vi "Move Menu Up.vi"(8 "error in (no error)":errorcluster, 11 "Display State In":T1={"Numeric"=0.0, "Array of Button References"=[], "Space Between Menu Buttons"=0, "Number of Menu Buttons"=0, "Array of Button Names"=[], "Most Recent Vertical Position"=0, "This VI"=refnum, "Current Action"=enum."Not Moving", "Most Recent Distance Traveled"=0, "Method"=enum."Move Up", "Data In"=0} caption="State") -> (0 "error out":errorcluster, 3 "Display State Out":T1={"Numeric"=0.0, "Array of Button References"=[], "Space Between Menu Buttons"=0, "Number of Menu Buttons"=0, "Array of Button Names"=[], "Most Recent Vertical Position"=0, "This VI"=refnum, "Current Action"=enum."Not Moving", "Most Recent Distance Traveled"=0, "Method"=enum."Move Up", "Data In"=0} caption="State")   [LabVIEW 2011, in "Sliding Menu Library.lvlib" / "Sliding Menu XControl.xctl"]
uses:
  Sliding Menu XControl.xctl
  Sliding Menu State.ctl
  Menu Button Library/Menu Button xControl/Menu Button xControl.xctl
  Sliding Menu SubVIs/Sliding Menu Type Definitions/Current User Action.ctl
  Sliding Menu Methods.ctl
  Sliding Menu Data.ctl
  Sliding Menu Library.lvlib
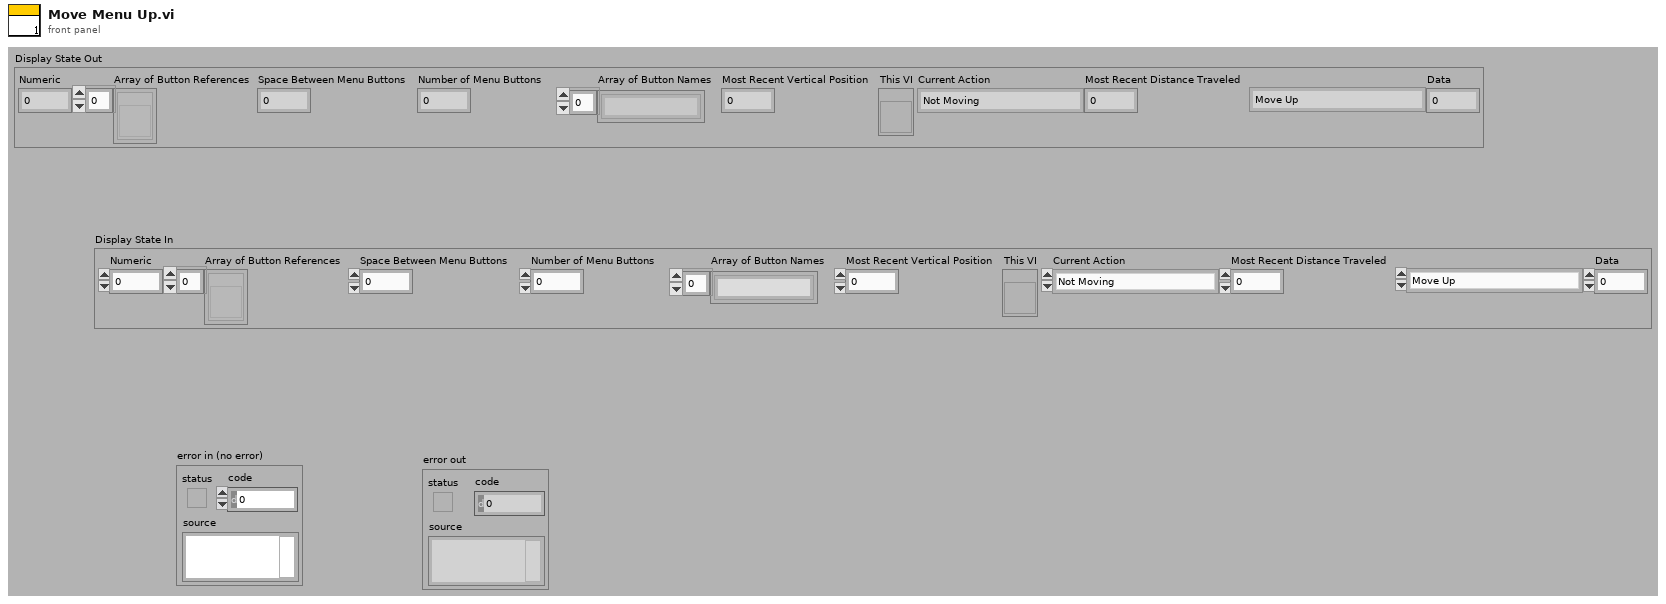
[diagram p1: front panel]
types:
  T1 = typedef "Sliding Menu Library.lvlib/Sliding Menu XControl.xctl/Sliding Menu State.ctl" = cluster{"Numeric":dbl, "Array of Button References":refnum<vi>[], "Space Between Menu Buttons":i32, "Number of Menu Buttons":i32, "Array of Button Names":string[], "Most Recent Vertical Position":i32, "This VI":refnum<vi>, "Current Action":T2, "Most Recent Distance Traveled":i32, "Method":T3, "Data In":T4}
  T2 = typedef "Sliding Menu Library.lvlib/Current User Action.ctl" = enum16{"Not Moving", "Mouse Down", "Mouse Up No Dragging", "Bounce Up Needed", "Bounce Down Needed", "Dragging", "Easing"}
  T3 = typedef "Sliding Menu Methods.ctl" = enum16{"Resize", "Move Up", "Move Down", "Move to 0"}
  T4 = typedef "Sliding Menu Library.lvlib/Sliding Menu XControl.xctl/Sliding Menu Data.ctl" = i32
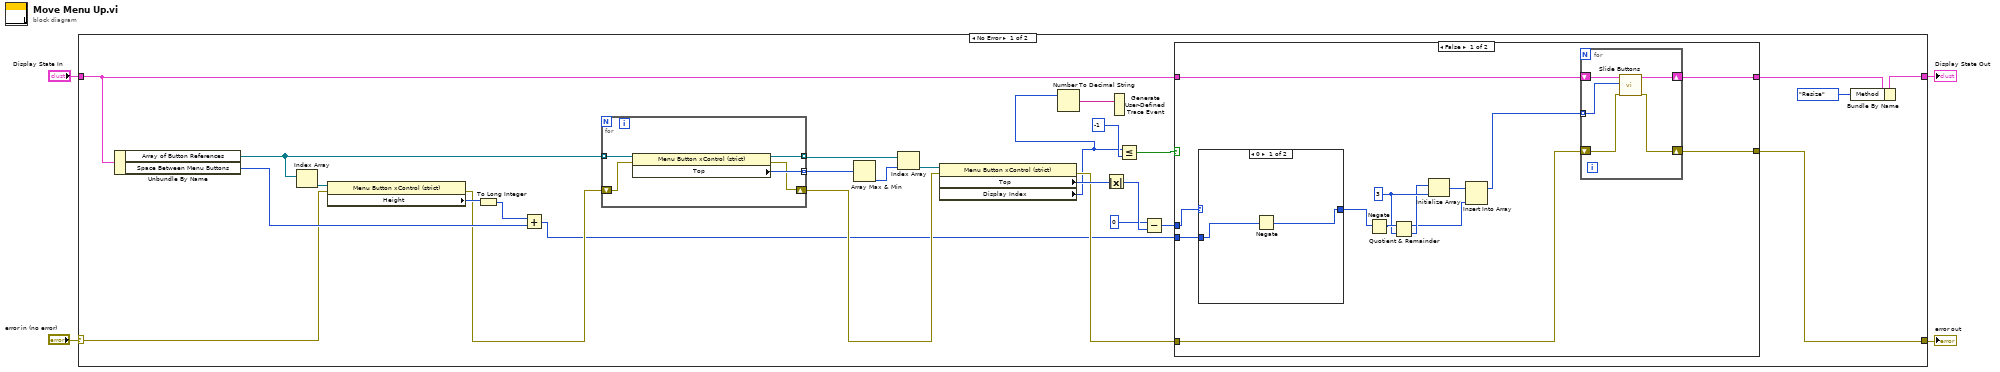
[diagram p0: block diagram]
diagram:
  n1 = case shown="No Error" "error in (no error)" {
    selector: "error in (no error)" -> [w16 w61]
    tunnel: [w12 w61] -> w1
    tunnel: "Display State In" -> [w28 w60]
    tunnel: [w30 w60] -> w2
    frame No Error {
      n2 = Unbundle By Name(w28) -> ("Array of Button References"=w24:refnum<vi>[], "Space Between Menu Buttons"=w19:i32)
      n3 = Index Array(array=w24) -> (element=w23:refnum<vi>)  [unwired: 1 in]
      n4 = property class="Menu Button xControl (strict)"(reference=w23, error in=w16) -> (error out=w15:errorcluster, "Height"=w18:u32)  [unwired: 1 out]
      n5 = To Long Integer(number=w18) -> (32bit integer=w17:i32)
      n6 = Add(x=w17, y=w19) -> (x+y=w9:i32)
      n7 = for {
        tunnel: w24 -> [w59] mode=indexing
        tunnel: [w58] -> w27 mode=indexing
        tunnel: [w57] -> w26 mode=indexing
        shift-right: [w56] -> w14
        shift-left: w15 -> [w55]
        n8 = property class="Menu Button xControl (strict)"(reference=w59, error in=w55) -> (reference out=w57:refnum<vi>, error out=w56:errorcluster, "Top"=w58:i32)
      }
      n9 = Array Max & Min(array=w27) -> (min index (indices)=w25:i32)  [unwired: 3 out]
      n10 = Index Array(array=w26, index=w25) -> (element=w22:refnum<vi>)
      n11 = property class="Menu Button xControl (strict)"(reference=w22, error in=w14) -> (error out=w13:errorcluster, "Top"=w21:i32, "Display Index"=w5:i32)  [unwired: 1 out]
      n12 = Number To Decimal String(number=w5) -> (decimal integer string=w6:string)  [unwired: 1 in]
      n13 = Absolute Value(x=w21) -> (abs(x)=w20:i32)
      n14 = Generate User-Defined Trace Event(2:w6) -> ()  [unwired: 1 in]
      n15 = Less Or Equal?(x=w5, y=-1 ("x")) -> (x <= y?=w7:bool)
      n16 = Subtract(x=0, y=w20) -> (x-y=w10:i32)
      n17 = case shown="False" w7 {
        tunnel: [w44 w54] -> w31
        tunnel: w28 -> [w43 w54]
        tunnel: w13 -> [w42 w53]
        tunnel: [w35 w53] -> w12
        tunnel: w10 -> [w34 _]
        tunnel: w9 -> [w32 _]
        frame False {
          w40 = 3 ("y")
          n18 = case shown="0" w34 {
            selector: w34 -> [_ w47]
            tunnel: [w45 w47] -> w33
            tunnel: w32 -> [w46 _]
            frame 0 {
              n19 = Negate(x=w46) -> (-x=w45:i32)
            }
            frame Default {
            }
          }
          n20 = Negate(x=w33) -> (-x=w41:i32)
          n21 = Quotient & Remainder(x=w41, y=w40) -> (x-y*floor(x/y)=w36:i32, floor(x/y)=w37:i32)
          n22 = Initialize Array(w37, w40) -> (w39:i32[])
          n23 = Insert Into Array(array=w39, new element=w36) -> (w38:i32[])  [unwired: 1 in]
          n24 = for {
            shift-right: [w51] -> w44
            shift-left: w43 -> [w50]
            shift-right: [w52] -> w35
            shift-left: w42 -> [w49]
            tunnel: w38 -> [w48] mode=indexing
            n25 = call "Slide Buttons.vi"("error in (no error)"=w49, "Distance"=w48, "Display State In"=w50) -> ("error out"=w52:errorcluster, "Display State Out"=w51:T1)  [unwired: 7 in]
          }
        }
        frame True {
          # "This checks to make sure you're not tyring to move lower\nthan you should"
        }
      }
      n26 = Bundle By Name(cluster=w31, "Method"=Sliding_Menu_Methods."Resize") -> (w30:T1)
    }
    frame Error {
    }
  }
  "error out" <- w1
  "Display State Out" <- w2
